vi "Draw Body_picture.vi"(8 "error in":errorcluster, 9 "picture":picture, 10 "Body Data":T2[](array[typedef]) {"LeanTrackingState" items=["NotTracked", "Inferred", "Tracked"]; "HandRightState" items=["Unknown", "NotTracked", "Open", "Closed", "Lasso"]; "HandRightConfidence" items=["Low", "High"]; "HandLeftState" items=["Unknown", "NotTracked", "Open", "Closed", "Lasso"]; "HandLeftConfidence" items=["Low", "High"]; "ClippedEdges" items=["None"=0, "Right"=1, "Left"=2, "Top"=4, "Bottom"=8]}, 11 "KinectSensor References":T1) -> (0 "error out":errorcluster, 1 "picture out":picture, 3 "KinectSensor References out":T1)   [LabVIEW 2014]
uses:
  controls/BodyData.ctl
  Microsoft.Kinect
  controls/KinectSensor References.ctl
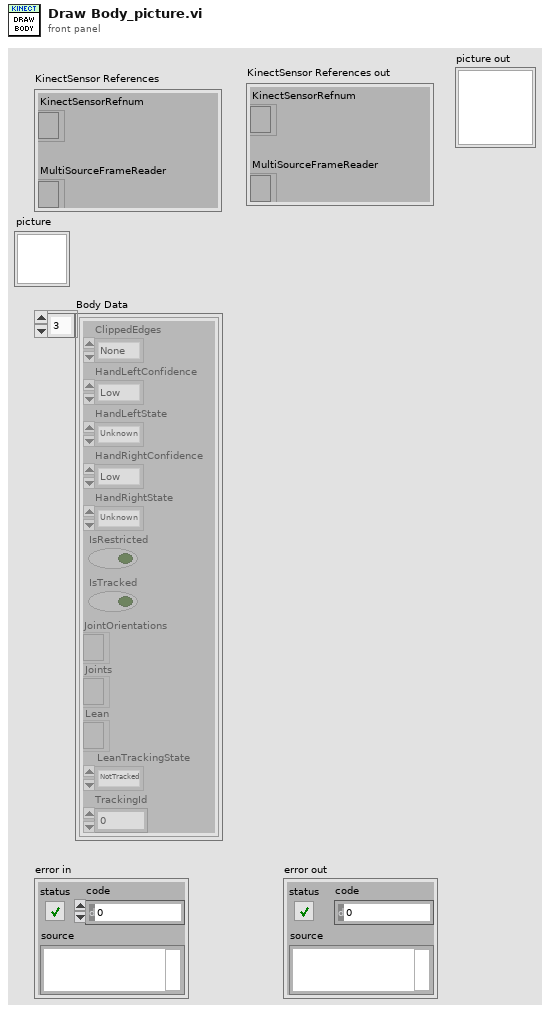
[diagram p1: front panel]
types:
  T1 = typedef "KinectSensor References.ctl" = cluster{"KinectSensorRefnum":refnum<k24>, "MultiSourceFrameReader":refnum<k24>}
  T2 = typedef "BodyData.ctl" = cluster{"ClippedEdges":i32, "HandLeftConfidence":i32, "HandLeftState":i32, "HandRightConfidence":i32, "HandRightState":i32, "IsRestricted":bool, "IsTracked":bool, "JointOrientations":refnum<k24>, "Joints":refnum<k24>, "Lean":refnum<k24>, "LeanTrackingState":i32, "TrackingId":u64}
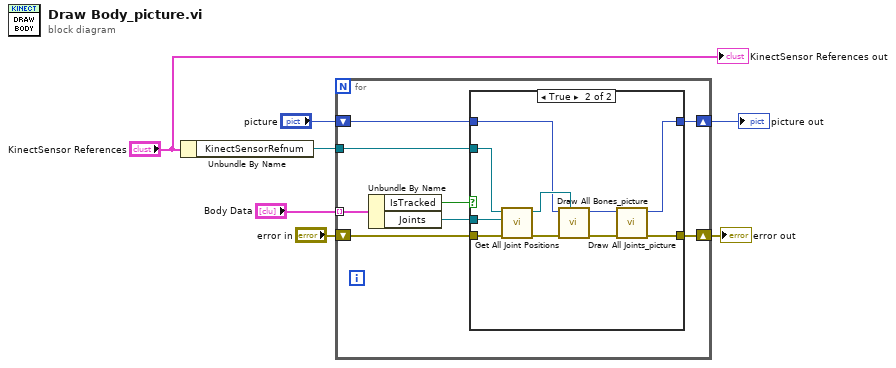
[diagram p0: block diagram]
diagram:
  n1 = Unbundle By Name("KinectSensor References") -> ("KinectSensorRefnum"=w5:refnum<k24>)
  n2 = for {
    tunnel: "Body Data" -> [w15] mode=indexing
    tunnel: w5 -> [w12]
    shift-right: [w11] -> w4
    shift-left: "error in" -> [w10]
    shift-right: [w9] -> w2
    shift-left: "picture" -> [w8]
    n3 = Unbundle By Name(w15) -> ("IsTracked"=w14:bool, "Joints"=w13:refnum<k24>)
    n4 = case shown="True" w14 {
      tunnel: w13 -> [_ w27]
      tunnel: w12 -> [_ w25]
      tunnel: [w17 w21] -> w11
      tunnel: w10 -> [w17 w24]
      tunnel: [w16 w20] -> w9
      tunnel: w8 -> [w16 w18]
      frame False {
      }
      frame True {
        n5 = call "Get All Joint Positions.vi"("error in (no error)"=w24, "Joints"=w27, "KinectSensor Reference"=w25) -> ("error out"=w26:errorcluster, "Joints"=w23:refnum<k24>)  [unwired: 7 in]
        n6 = call "Draw All Bones_picture.vi"("Joints"=w23, "error in"=w26, "picture"=w18) -> ("error out"=w22:errorcluster, "picture out"=w19:picture)  [unwired: 7 in]
        n7 = call "Draw All Joints_picture.vi"("error out"=w22, "picture"=w19) -> ("error out 2"=w21:errorcluster, "picture out"=w20:picture)  [unwired: 8 in]
      }
    }
  }
  "error out" <- w4
  "picture out" <- w2
  "KinectSensor References out" <- "KinectSensor References"
